vi "bofxy.vi"(5 "tilt_y":dbl, 7 "tilt_x":dbl, 10 "Y":dbl[](array[numeric]) format="%#_13g", 11 "X":dbl[](array[numeric]) format="%#_13g") -> (1 "dB dy":T1, 2 "dB dx":T2, 3 "B":cluster{"Bx":dbl[], "By":dbl[], "Bz":dbl[]})   [LabVIEW 2017]
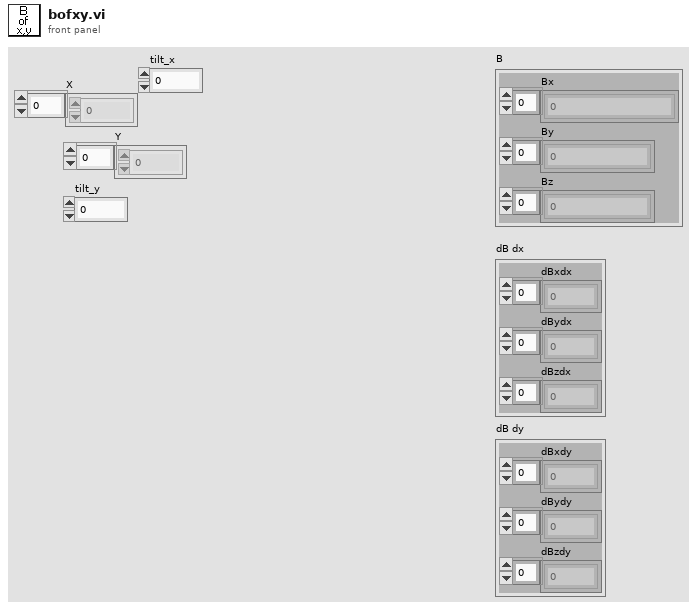
[diagram p1: front panel]
types:
  T1 = cluster{"dBxdy":dbl[], "dBydy":dbl[], "dBzdy":dbl[]}
  T2 = cluster{"dBxdx":dbl[], "dBydx":dbl[], "dBzdx":dbl[]}
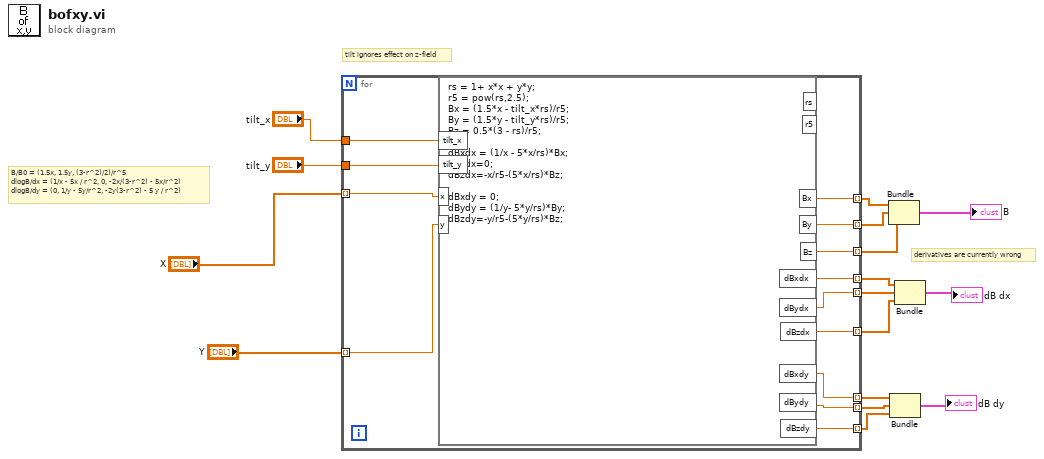
[diagram p0: block diagram]
diagram:
  # "derivatives are currently wrong"
  # "tilt ignores effect on z-field"
  # "B/B0 = (1.5x, 1.5y, (3-r^2)/2)/r^5\ndlogB/dx = (1/x - 5x / r^2, 0, -2x/(3-r^2) - 5x/r^2)\ndlogB/dy = (0, 1/y - 5y/r^2, -2y(3-r^2) - 5 y / r^2)"
  n1 = for {
    tunnel: [w29] -> w15 mode=indexing
    tunnel: [w28] -> w14 mode=indexing
    tunnel: [w27] -> w13 mode=indexing
    tunnel: [w26] -> w12 mode=indexing
    tunnel: [w25] -> w11 mode=indexing
    tunnel: [w24] -> w10 mode=indexing
    tunnel: [w23] -> w9 mode=indexing
    tunnel: [w22] -> w8 mode=indexing
    tunnel: [w21] -> w7 mode=indexing
    tunnel: "X" -> [w20] mode=indexing
    tunnel: "Y" -> [w19] mode=indexing
    tunnel: "tilt_x" -> [w18]
    tunnel: "tilt_y" -> [w17]
    n2 = formula code="rs = 1+ x*x + y*y;\nr5 = pow(rs,2.5);\nBx = (1.5*x - tilt_x*rs)/r5;\nBy = (1.5*y - tilt_y*rs)/r5;\nBz = 0.5*(3 - rs)/r5;\n\ndBxdx = (1/x - 5*x/rs)*Bx;\ndBydx=0;\ndBzdx=-x/r5-(5*x/rs)*Bz;\n\ndBxdy = 0;\ndBydy = (1/y- 5*y/rs)*By;\ndBzdy=-y/r5-(5*y/rs)*Bz;"("x"=w20, "y"=w19, "tilt_x"=w18, "tilt_y"=w17) -> ("Bx"=w29:dbl, "By"=w28:dbl, "Bz"=w27:dbl, "dBxdx"=w26:dbl, "dBydx"=w25:dbl, "dBzdx"=w24:dbl, "dBxdy"=w23:dbl, "dBydy"=w22:dbl, "dBzdy"=w21:dbl)  [unwired: 2 out]
  }
  n3 = Bundle(w15, w14, w13) -> (→"B":cluster{dbl[], dbl[], dbl[]})  [unwired: 1 in]
  n4 = Bundle(w9, w8, w7) -> (→"dB dy":cluster{dbl[], dbl[], dbl[]})  [unwired: 1 in]
  n5 = Bundle(w12, w11, w10) -> (→"dB dx":cluster{dbl[], dbl[], dbl[]})  [unwired: 1 in]
